vi "AlliGator Get Temp Accumulated File Name.vi"(8 "error in (no error)":errorcluster, 9 "Averaged?":bool, 11 "Time-Series Folder":path) -> (0 "error out":errorcluster, 2 "filename without extension":string, 3 "temporary file name":path)   [LabVIEW 2021, in "AlliGator Accumulated Dataset.lvlib"]
doc: "Builds name of acccumulated or averaged dataset displayed in AlliGator's title bar."
uses:
  AlliGator Accumulated Dataset.lvlib
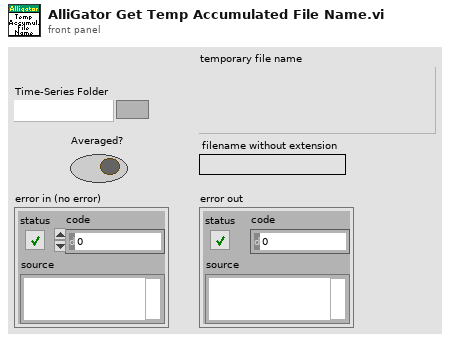
[diagram p1: front panel]
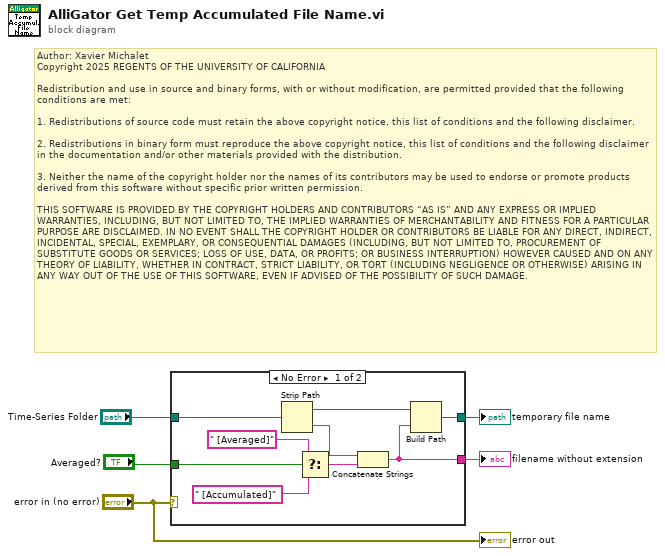
[diagram p0: block diagram]
diagram:
  # "Author: Xavier Michalet\nCopyright 2025 REGENTS OF THE UNIVERSITY OF CALIFORNIA\n\nRedistribution and use in source and binary forms, with or without modification, are permitted provided that the following conditions are met:\n\n1. Redistributions of source code must retain the above copyright notice, this list of conditions and the following disclaimer.\n\n2. Redistributions in binary form must reproduce the above copyright notice, this list of conditions and the following disclaimer in the documentation and/or other materials provided with the distribution.\n\n3. Neither the name of the copyright holder nor the names of its contributors may be used to endorse or promote products derived from this software without specific prior written permission.\n\nTHIS SOFTWARE IS PROVIDED BY THE COPYRIGHT HOLDERS AND CONTRIBUTORS “AS IS” AND ANY EXPRESS OR IMPLIED WARRANTIES, INCLUDING, BUT NOT LIMITED TO, THE IMPLIED WARRANTIES OF MERCHANTABILITY AND FITNESS FOR A PARTICULAR PURPOSE ARE DISCLAIMED. IN NO EVENT SHALL THE COPYRIGHT HOLDER OR CONTRIBUTORS BE LIABLE FOR ANY DIRECT, INDIRECT, INCIDENTAL, SPECIAL, EXEMPLARY, OR CONSEQUENTIAL DAMAGES (INCLUDING, BUT NOT LIMITED TO, PROCUREMENT OF SUBSTITUTE GOODS OR SERVICES; LOSS OF USE, DATA, OR PROFITS; OR BUSINESS INTERRUPTION) HOWEVER CAUSED AND ON ANY THEORY OF LIABILITY, WHETHER IN CONTRACT, STRICT LIABILITY, OR TORT (INCLUDING NEGLIGENCE OR OTHERWISE) ARISING IN ANY WAY OUT OF THE USE OF THIS SOFTWARE, EVEN IF ADVISED OF THE POSSIBILITY OF SUCH DAMAGE."
  n1 = case shown="No Error" "error in (no error)" {
    tunnel: [w13 w15] -> w5
    tunnel: [w12 _] -> w4
    tunnel: "Averaged?" -> [w11 _]
    tunnel: "Time-Series Folder" -> [w7 w15]
    frame No Error {
      n2 = Strip Path(path=w7) -> (stripped path=w14:path, name=w6:string)
      n3 = Select(t=" [Averaged]" ("string"), s=w11, f=" [Accumulated]" ("string")) -> (s? t:f=w9:string)
      n4 = Concatenate Strings(w6, w9) -> (w12:string)
      n5 = Build Path(base path=w14, name or relative path=w12) -> (appended path=w13:path)
    }
    frame Error {
    }
  }
  "temporary file name" <- w5
  "filename without extension" <- w4
  "error out" <- "error in (no error)"
